vi "GuiUpdate.vi"(7 "GuiRef":T1, 8 "error in":errorcluster, 9 "States":T2=enum."PostUUT") -> (0 "error out":errorcluster, 1 "GuiRefOut":T1, 2 "PASS/FAIL":bool)   [LabVIEW 2013]
uses:
  Ctl/States.ctl
  Ctl/LEDState.ctl
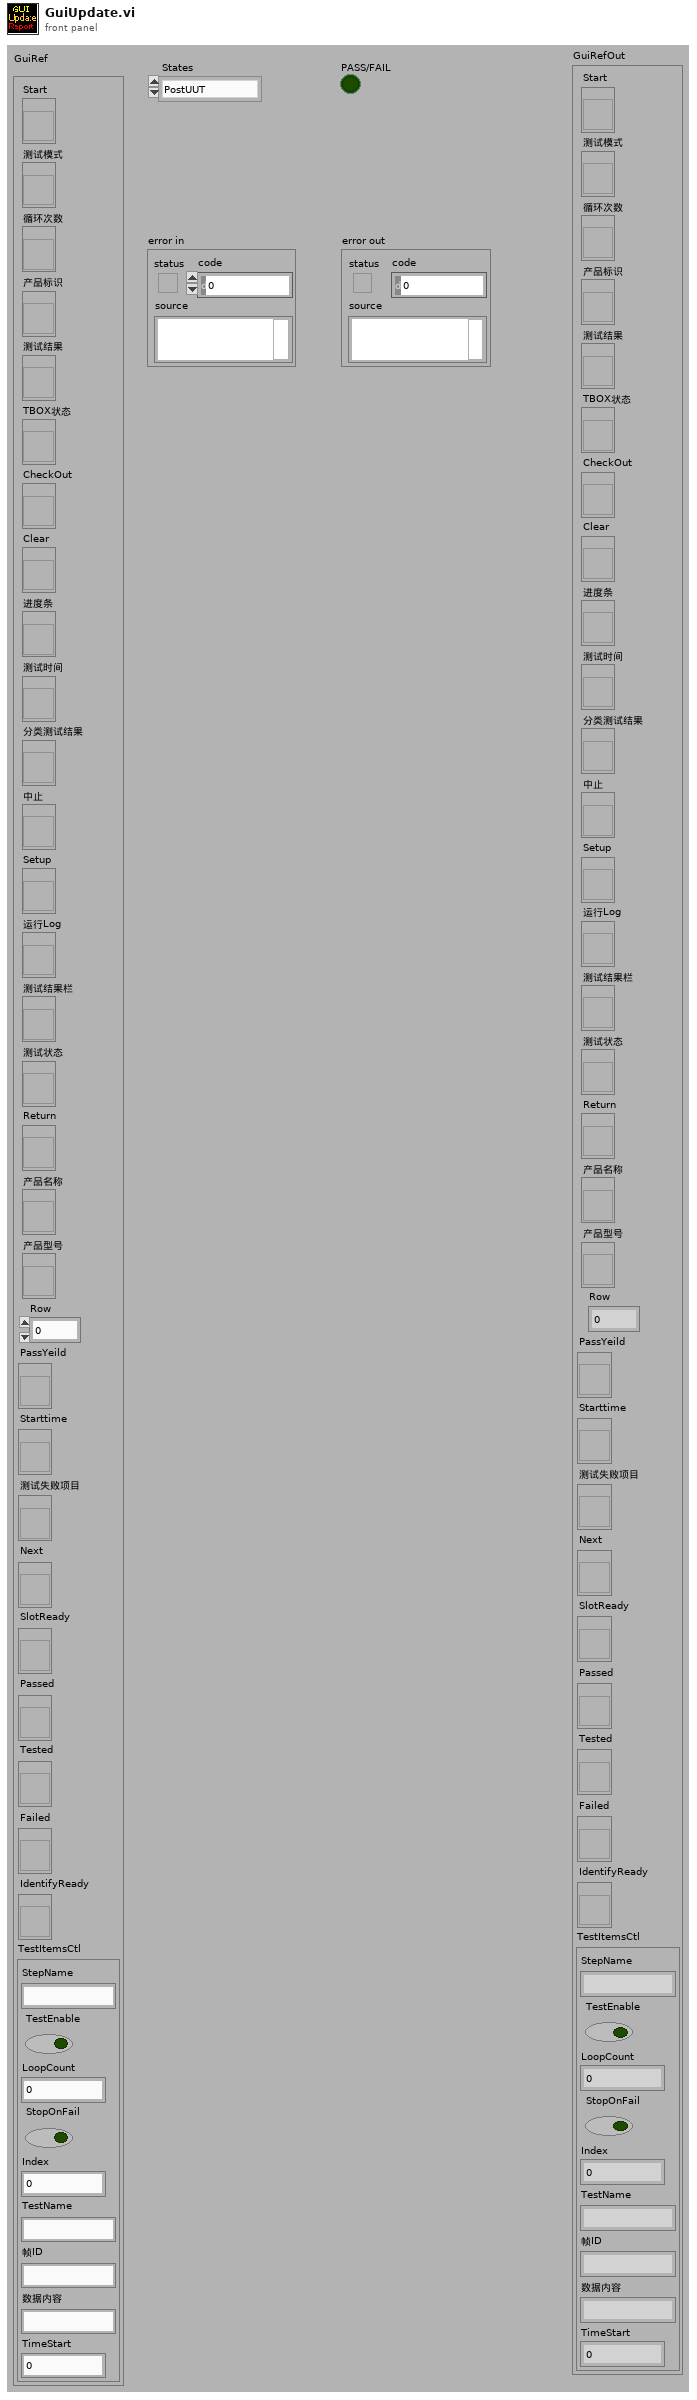
[diagram p1: front panel]
types:
  T1 = typedef "控件.ctl" = cluster{"Start":refnum<vi>, "测试模式":refnum<vi>, "循环次数":refnum<vi>, "产品标识":refnum<vi>, "测试结果":refnum<vi>, "TBOX状态":refnum<vi>, "CheckOut":refnum<vi>, "Clear":refnum<vi>, "进度条":refnum<vi>, "测试时间":refnum<vi>, "分类测试结果":refnum<vi>, "中止":refnum<vi>, "Setup":refnum<vi>, "运行Log":refnum<vi>, "测试结果栏":refnum<vi>, "测试状态":refnum<vi>, "Return":refnum<vi>, "产品名称":refnum<vi>, "产品型号":refnum<vi>, "Row":i32, "PassYeild":refnum<vi>, "Starttime":refnum<vi>, "测试失败项目":refnum<vi>, "Next":refnum<vi>, "SlotReady":refnum<vi>, "Passed":refnum<vi>, "Tested":refnum<vi>, "Failed":refnum<vi>, "IdentifyReady":refnum<vi>, "TestItemsCtl":cluster{"StepName":string, "TestEnable":bool, "LoopCount":u32, "StopOnFail":bool, "Index":u32, "TestName":string, "帧ID":string, "数据内容":string, "TimeStart":u32}}
  T2 = typedef "States.ctl" = enum16{"Init", "PreUUT", "Idle", "SetUp", "TestSequence", "PostUUT", "StopTest", "Debug Mode", "Selection Mode", "Loop Mode", "Error", "Wait"}
  T3 = enum8{"Enabled", "Disabled", "Disabled and Grayed Out"}
  T4 = typedef "LEDState.ctl" = enum16{"默认", "闪烁", "停止闪烁", "真", "假"}
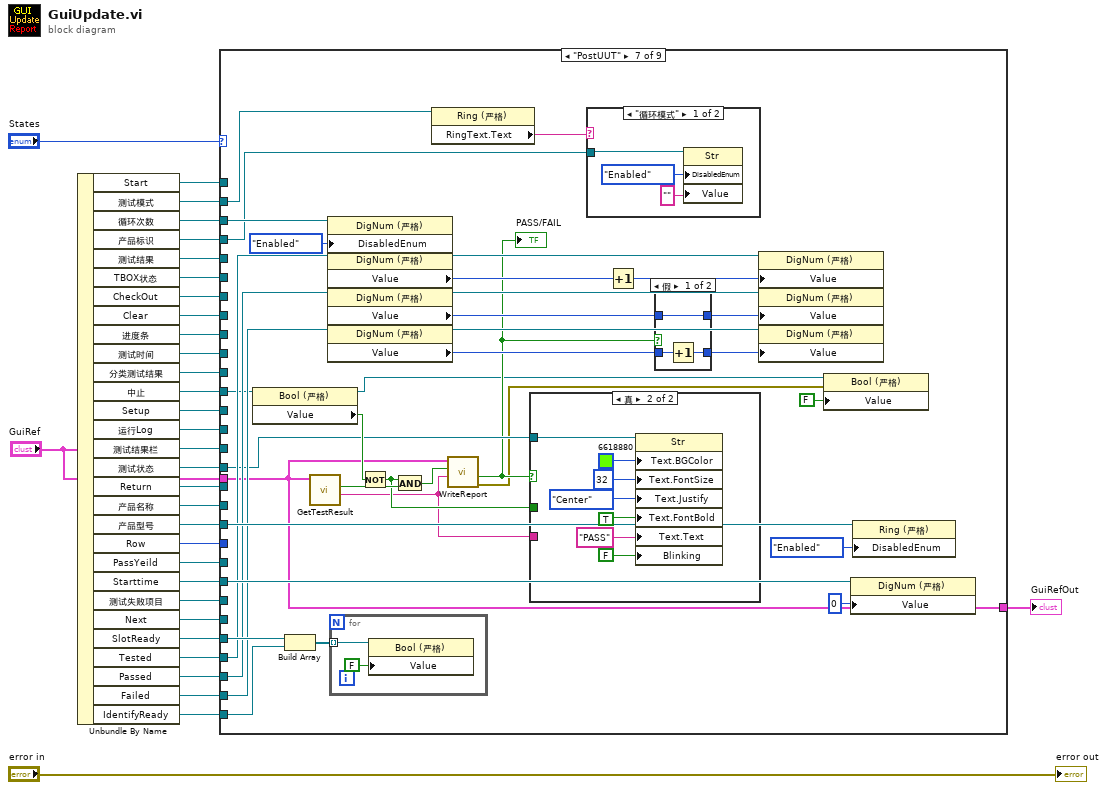
[diagram p0: block diagram]
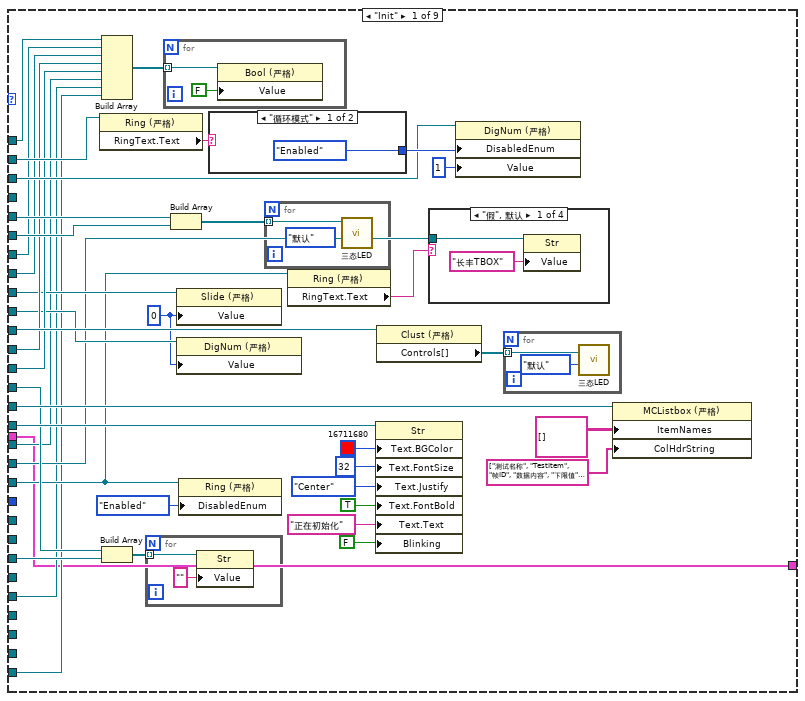
[diagram p2: hidden frame]
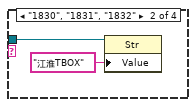
[diagram p3: hidden frame]
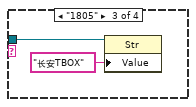
[diagram p4: hidden frame]
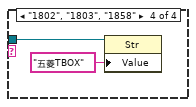
[diagram p5: hidden frame]
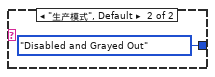
[diagram p6: hidden frame]
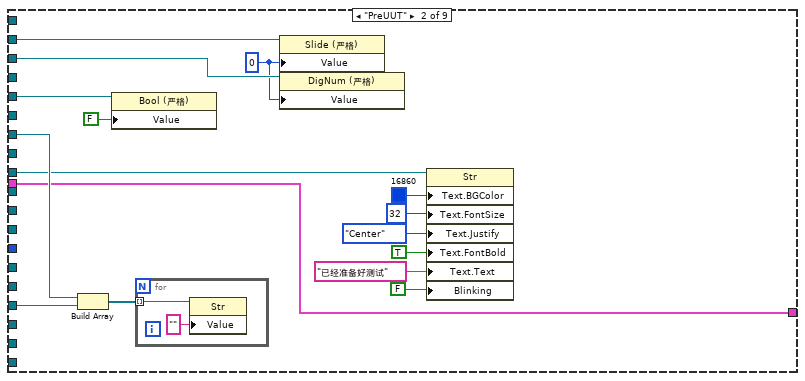
[diagram p7: hidden frame]
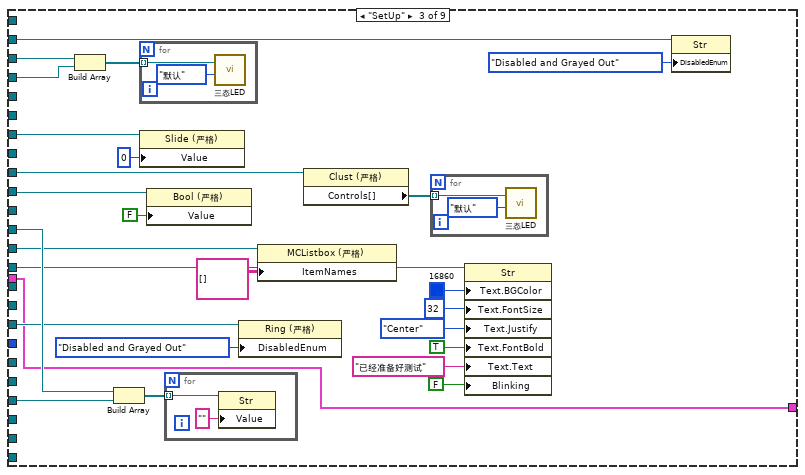
[diagram p8: hidden frame]
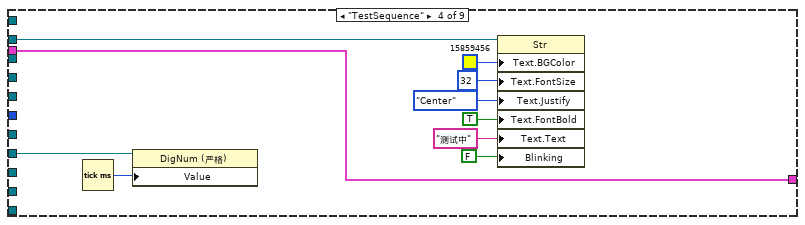
[diagram p9: hidden frame]
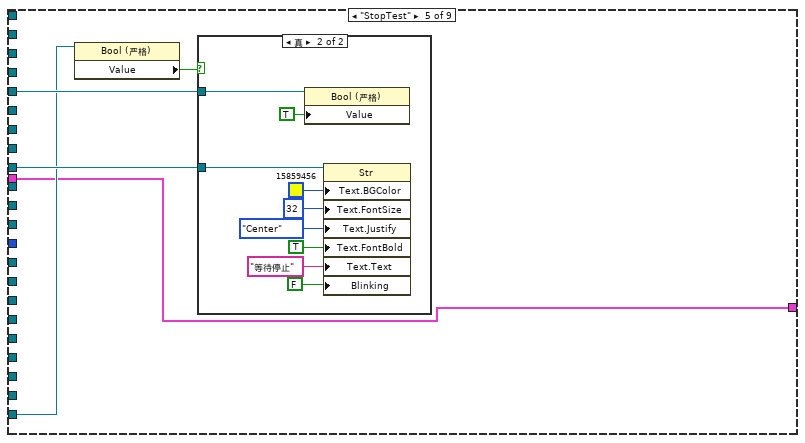
[diagram p10: hidden frame]
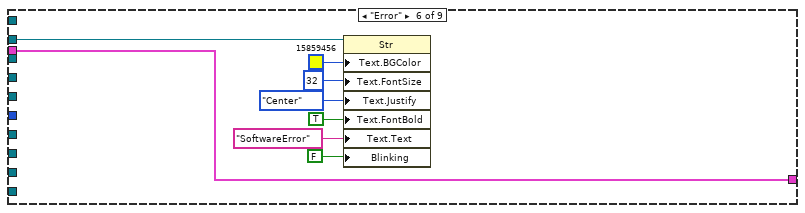
[diagram p12: hidden frame]
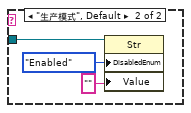
[diagram p13: hidden frame]
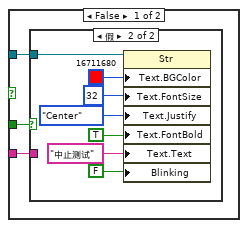
[diagram p14: hidden frame]
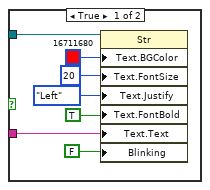
[diagram p15: hidden frame]
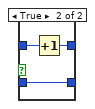
[diagram p16: hidden frame]
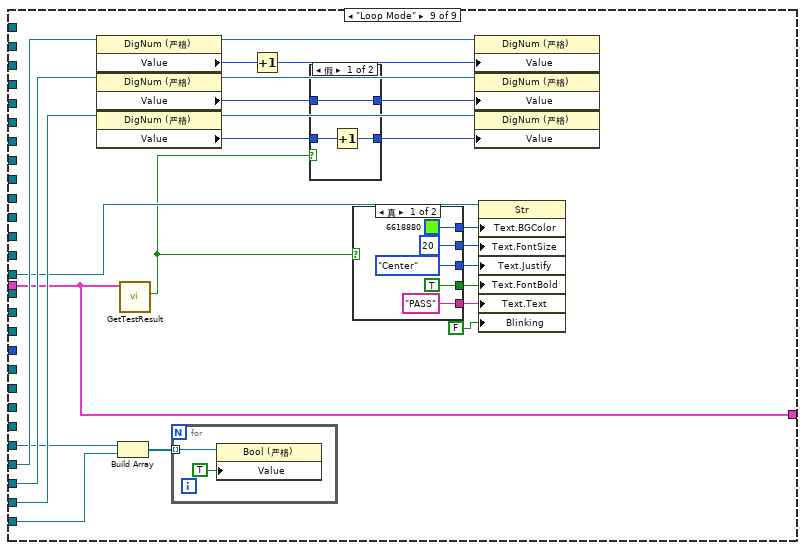
[diagram p18: hidden frame]
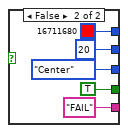
[diagram p19: hidden frame]
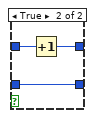
[diagram p20: hidden frame]
diagram:
  n1 = Unbundle By Name("GuiRef") -> ("Start"=w31:refnum<vi>, "测试模式"=w30:refnum<vi>, "循环次数"=w29:refnum<vi>, "产品标识"=w28:refnum<vi>, "测试结果"=w27:refnum<vi>, "TBOX状态"=w26:refnum<vi>, "CheckOut"=w25:refnum<vi>, "Clear"=w24:refnum<vi>, "进度条"=w23:refnum<vi>, "测试时间"=w22:refnum<vi>, "分类测试结果"=w21:refnum<vi>, "中止"=w2:refnum<vi>, "Setup"=w20:refnum<vi>, "运行Log"=w19:refnum<vi>, "测试结果栏"=w18:refnum<vi>, "测试状态"=w17:refnum<vi>, "Return"=w16:refnum<vi>, "产品名称"=w15:refnum<vi>, "产品型号"=w14:refnum<vi>, "Row"=w13:i32, "PassYeild"=w12:refnum<vi>, "Starttime"=w11:refnum<vi>, "测试失败项目"=w10:refnum<vi>, "Next"=w9:refnum<vi>, "SlotReady"=w8:refnum<vi>, "Tested"=w7:refnum<vi>, "Passed"=w6:refnum<vi>, "Failed"=w5:refnum<vi>, "IdentifyReady"=w3:refnum<vi>)
  n2 = case shown="\"PostUUT\"" "States" {
    tunnel: w31 -> [w63 _ _ _ _ _ _ _ _]
    tunnel: w30 -> [w73 _ _ _ _ _ w180 _ _]
    tunnel: w29 -> [w70 _ _ _ _ _ w208 _ _]
    tunnel: w28 -> [_ _ w123 _ _ _ w178 _ _]
    tunnel: w27 -> [w66 _ w115 _ _ _ _ _ _]
    tunnel: w26 -> [w65 _ w114 _ _ _ _ _ _]
    tunnel: w25 -> [w62 _ _ _ _ _ _ _ _]
    tunnel: w24 -> [w61 _ _ _ _ _ _ _ _]
    tunnel: w23 -> [w57 w95 w119 _ _ _ _ _ _]
    tunnel: w22 -> [w56 w94 _ _ _ _ _ _ _]
    tunnel: w21 -> [w68 _ w116 _ _ _ _ _ _]
    tunnel: w20 -> [w59 _ _ _ _ _ _ _ _]
    tunnel: w19 -> [w44 w107 w133 _ _ _ _ _ _]
    tunnel: w18 -> [w54 _ w121 _ _ _ _ _ _]
    tunnel: w17 -> [w51 w98 w126 w145 w155 w167 w187 _ w255]
    tunnel: w16 -> [w35 _ _ _ _ _ _ _ _]
    tunnel: w15 -> [w40 _ _ _ _ _ _ _ _]
    tunnel: w14 -> [w39 _ w124 _ _ _ w204 _ _]
    tunnel: w13 -> [_ _ _ _ _ _ _ _ _]
    tunnel: w12 -> [_ _ _ _ _ _ _ _ _]
    tunnel: w11 -> [_ _ _ w144 _ _ w206 _ _]
    tunnel: w10 -> [w43 w106 w134 _ _ _ _ _ _]
    tunnel: w9 -> [_ _ _ _ _ _ _ _ _]
    tunnel: w8 -> [w37 _ _ _ _ _ w209 _ w252]
    tunnel: w7 -> [_ _ _ _ _ _ w202 _ w272]
    tunnel: w6 -> [_ _ _ _ _ _ w201 _ w259]
    tunnel: w5 -> [_ _ _ _ _ _ w200 _ w258]
    tunnel: "GuiRef" -> [w34 w92 w110 w142 w152 w166 w174 w248 w249]
    tunnel: w3 -> [w36 _ _ _ w153 _ w176 _ w250]
    tunnel: w2 -> [w60 w97 w112 _ w156 _ w175 _ _]
    tunnel: [w34 w92 w110 w142 w152 w166 w174 w248 w249] -> w1
    frame "Init" {
      w55 = 0 ("值")
      n3 = property class="Ring (严格)"(reference=w73) -> ("RingText.Text"=w72:string)  [unwired: 1 in, 2 out]
      n4 = Build Array(w63, w62, w61, w60, w59, w35, w37, w36) -> (w58:refnum<vi>[])
      n5 = Build Array(w44, w43) -> (w42:refnum<vi>[])
      n6 = for {
        tunnel: w42 -> [w83] mode=indexing
        n7 = property class="Str"(reference=w83, "Value"="" ("值")) -> ()  [unwired: 1 in, 2 out]
      }
      n8 = for {
        tunnel: w58 -> [w84] mode=indexing
        n9 = property class="Bool (严格)"(reference=w84, "Value"=FALSE) -> ()  [unwired: 1 in, 2 out]
      }
      n10 = Build Array(w66, w65) -> (w64:refnum<vi>[])
      n11 = property class="Slide (严格)"(reference=w57, "Value"=w55) -> ()  [unwired: 1 in, 2 out]
      n12 = property class="DigNum (严格)"(reference=w56, "Value"=w55) -> ()  [unwired: 1 in, 2 out]
      n13 = property class="Ring (严格)"(reference=w39, "DisabledEnum"=T3."Enabled" ("禁用")) -> ()  [unwired: 1 in, 2 out]
      n14 = case shown="\"循环模式\"" w72 {
        tunnel: [T3."Enabled" ("禁用") T3."Disabled and Grayed Out" ("禁用")] -> w71
        frame "循环模式" {
        }
        frame "生产模式", Default {
        }
      }
      n15 = for {
        tunnel: w64 -> [w86] mode=indexing
        n16 = call "三态LED.vi"("State"=LEDState."默认", "Ctl引用句柄"=w86) -> ()  [unwired: 4 in, 2 out]
      }
      n17 = property class="Ring (严格)"(reference=w39) -> ("RingText.Text"=w38:string)  [unwired: 1 in, 2 out]
      n18 = property class="Str"(reference=w51, "Text.BGColor"=u32 16711680, "Text.FontSize"=32 ("值"), "Text.Justify"=enum16{"Left", "Center", "Right"}."Center" ("文本.调整"), "Text.FontBold"=TRUE ("文本.字体:粗体"), "Text.Text"="正在初始化" ("文本.文本"), "Blinking"=FALSE ("文本.字体:粗体")) -> ()  [unwired: 1 in, 2 out]
      n19 = property class="Clust (严格)"(reference=w68) -> ("Controls[]"=w67:refnum<vi>[])  [unwired: 1 in, 2 out]
      n20 = case shown="\"假\", 默认" w38 {
        tunnel: w40 -> [w74 w77 w79 w81]
        frame "假", Default {
          n21 = property class="Str"(reference=w74, "Value"="长丰TBOX" ("值")) -> ()  [unwired: 1 in, 2 out]
        }
        frame "1830", "1831", "1832" {
          n22 = property class="Str"(reference=w77, "Value"="江淮TBOX" ("值")) -> ()  [unwired: 1 in, 2 out]
        }
        frame "1805" {
          n23 = property class="Str"(reference=w79, "Value"="长安TBOX" ("值")) -> ()  [unwired: 1 in, 2 out]
        }
        frame "1802", "1803", "1858" {
          n24 = property class="Str"(reference=w81, "Value"="五菱TBOX" ("值")) -> ()  [unwired: 1 in, 2 out]
        }
      }
      n25 = property class="DigNum (严格)"(reference=w70, "DisabledEnum"=w71, "Value"=u32 1 ("值")) -> ()  [unwired: 1 in, 2 out]
      n26 = for {
        tunnel: w67 -> [w88] mode=indexing
        n27 = call "三态LED.vi"("State"=LEDState."默认", "Ctl引用句柄"=w88) -> ()  [unwired: 4 in, 2 out]
      }
      n28 = property class="MCListbox (严格)"(reference=w54, "ItemNames"=string[][] [] ("项名"), "ColHdrString"=string[] ["测试名称", "TestItem", "帧ID", "数据内容", "下限值", "上限值", "单位", "间隔时间", "测量值", "结果", "测试时间", "备注", "测试项目"] ("列首字符串[]")) -> ()  [unwired: 1 in, 2 out]
    }
    frame "PreUUT" {
      w93 = 0
      n29 = Build Array(w107, w106) -> (w105:refnum<vi>[])
      n30 = property class="Bool (严格)"(reference=w97, "Value"=FALSE ("值")) -> ()  [unwired: 1 in, 2 out]
      n31 = for {
        tunnel: w105 -> [w109] mode=indexing
        n32 = property class="Str"(reference=w109, "Value"="" ("值")) -> ()  [unwired: 1 in, 2 out]
      }
      n33 = property class="Slide (严格)"(reference=w95, "Value"=w93) -> ()  [unwired: 1 in, 2 out]
      n34 = property class="DigNum (严格)"(reference=w94, "Value"=w93) -> ()  [unwired: 1 in, 2 out]
      n35 = property class="Str"(reference=w98, "Text.BGColor"=u32 16860, "Text.FontSize"=32 ("值"), "Text.Justify"=enum16{"Left", "Center", "Right"}."Center" ("文本.调整"), "Text.FontBold"=TRUE ("文本.字体:粗体"), "Text.Text"="已经准备好测试" ("文本.文本"), "Blinking"=FALSE ("文本.字体:粗体")) -> ()  [unwired: 1 in, 2 out]
    }
    frame "SetUp" {
      n36 = Build Array(w115, w114) -> (w113:refnum<vi>[])
      n37 = Build Array(w133, w134) -> (w135:refnum<vi>[])
      n38 = for {
        tunnel: w113 -> [w136] mode=indexing
        n39 = call "三态LED.vi"("State"=LEDState."默认", "Ctl引用句柄"=w136) -> ()  [unwired: 4 in, 2 out]
      }
      n40 = property class="Slide (严格)"(reference=w119, "Value"=0 ("值")) -> ()  [unwired: 1 in, 2 out]
      n41 = property class="Bool (严格)"(reference=w112, "Value"=FALSE ("值")) -> ()  [unwired: 1 in, 2 out]
      n42 = for {
        tunnel: w135 -> [w141] mode=indexing
        n43 = property class="Str"(reference=w141, "Value"="" ("值")) -> ()  [unwired: 1 in, 2 out]
      }
      n44 = property class="Ring (严格)"(reference=w124, "DisabledEnum"=T3."Disabled and Grayed Out" ("禁用")) -> ()  [unwired: 1 in, 2 out]
      n45 = property class="MCListbox (严格)"(reference=w121, "ItemNames"=string[][] [] ("项名")) -> ()  [unwired: 1 in, 2 out]
      n46 = property class="Clust (严格)"(reference=w116) -> ("Controls[]"=w117:refnum<vi>[])  [unwired: 1 in, 2 out]
      n47 = for {
        tunnel: w117 -> [w138] mode=indexing
        n48 = call "三态LED.vi"("State"=LEDState."默认", "Ctl引用句柄"=w138) -> ()  [unwired: 4 in, 2 out]
      }
      n49 = property class="Str"(reference=w126, "Text.BGColor"=u32 16860, "Text.FontSize"=32 ("值"), "Text.Justify"=enum16{"Left", "Center", "Right"}."Center" ("文本.调整"), "Text.FontBold"=TRUE ("文本.字体:粗体"), "Text.Text"="已经准备好测试" ("文本.文本"), "Blinking"=FALSE ("文本.字体:粗体")) -> ()  [unwired: 1 in, 2 out]
      n50 = property class="Str"(reference=w123, "DisabledEnum"=T3."Disabled and Grayed Out" ("禁用")) -> ()  [unwired: 1 in, 2 out]
    }
    frame "TestSequence" {
      n51 = Tick Count (ms)() -> (millisecond timer value=w143:u32)
      n52 = property class="DigNum (严格)"(reference=w144, "Value"=w143) -> ()  [unwired: 1 in, 2 out]
      n53 = property class="Str"(reference=w145, "Text.BGColor"=u32 15859456, "Text.FontSize"=32 ("值"), "Text.Justify"=enum16{"Left", "Center", "Right"}."Center" ("文本.调整"), "Text.FontBold"=TRUE ("文本.字体:粗体"), "Text.Text"="测试中" ("文本.文本"), "Blinking"=FALSE ("文本.字体:粗体")) -> ()  [unwired: 1 in, 2 out]
    }
    frame "StopTest" {
      n54 = property class="Bool (严格)"(reference=w153) -> ("Value"=w154:bool)  [unwired: 1 in, 2 out]
      n55 = case shown="真" w154 {
        tunnel: w156 -> [_ w165]
        tunnel: w155 -> [_ w157]
        frame False {
        }
        frame True {
          n56 = property class="Bool (严格)"(reference=w165, "Value"=TRUE) -> ()  [unwired: 1 in, 2 out]
          n57 = property class="Str"(reference=w157, "Text.BGColor"=u32 15859456, "Text.FontSize"=32 ("值"), "Text.Justify"=enum16{"Left", "Center", "Right"}."Center" ("文本.调整"), "Text.FontBold"=TRUE ("文本.字体:粗体"), "Text.Text"="等待停止" ("文本.文本"), "Blinking"=FALSE ("文本.字体:粗体")) -> ()  [unwired: 1 in, 2 out]
        }
      }
    }
    frame "Error" {
      n58 = property class="Str"(reference=w167, "Text.BGColor"=u32 15859456, "Text.FontSize"=32 ("值"), "Text.Justify"=enum16{"Left", "Center", "Right"}."Center" ("文本.调整"), "Text.FontBold"=TRUE ("文本.字体:粗体"), "Text.Text"="SoftwareError" ("文本.文本"), "Blinking"=FALSE ("文本.字体:粗体")) -> ()  [unwired: 1 in, 2 out]
    }
    frame "PostUUT" {
      n59 = property class="Bool (严格)"(reference=w175) -> (reference out=w182:refnum<vi>, "Value"=w189:bool)  [unwired: 1 in, 1 out]
      n60 = Build Array(w209, w176) -> (w177:refnum<vi>[])
      n61 = call "GetTestResult.vi"("GuiRef"=w174) -> ("FailStep"=w184:string, "PASS/FAIL"=w190:bool)  [unwired: 9 in]
      n62 = property class="DigNum (严格)"(reference=w208, "DisabledEnum"=T3."Enabled" ("禁用")) -> ()  [unwired: 1 in, 2 out]
      n63 = property class="DigNum (严格)"(reference=w202) -> (reference out=w197:refnum<vi>, "Value"=w199:u32)  [unwired: 1 in, 1 out]
      n64 = property class="DigNum (严格)"(reference=w201) -> (reference out=w191:refnum<vi>, "Value"=w196:u32)  [unwired: 1 in, 1 out]
      n65 = property class="DigNum (严格)"(reference=w200) -> (reference out=w192:refnum<vi>, "Value"=w194:u32)  [unwired: 1 in, 1 out]
      n66 = for {
        tunnel: w177 -> [w211] mode=indexing
        n67 = property class="Bool (严格)"(reference=w211, "Value"=FALSE ("值")) -> ()  [unwired: 1 in, 2 out]
      }
      n68 = Not(x=w189) -> (.not. x?=w185:bool)
      n69 = And(x=w185, y=w190) -> (x .and. y?=w188:bool)
      n70 = property class="Ring (严格)"(reference=w180) -> ("RingText.Text"=w179:string)  [unwired: 1 in, 2 out]
      n71 = call "WriteReport.vi"("StepName"=w184, "Pass/Fail"=w188, "输出簇"=w174) -> ("error out"=w183:errorcluster, "DBresult"=w186:bool)  [unwired: 7 in]
      "PASS/FAIL" <- w186
      n72 = case shown="真" w186 {
        tunnel: w187 -> [w220 w241]
        tunnel: w185 -> [w219 _]
        tunnel: w184 -> [w218 _]
        frame False {
          n73 = case shown="假" w219 {
            tunnel: w220 -> [w222 w229]
            tunnel: w218 -> [w221 _]
            frame True {
              n74 = property class="Str"(reference=w222, "Text.BGColor"=u32 16711680, "Text.FontSize"=20 ("值"), "Text.Justify"=enum16{"Left", "Center", "Right"}."Left" ("文本.调整"), "Text.FontBold"=TRUE ("文本.字体:粗体"), "Text.Text"=w221, "Blinking"=FALSE ("文本.字体:粗体")) -> ()  [unwired: 1 in, 2 out]
            }
            frame False {
              n75 = property class="Str"(reference=w229, "Text.BGColor"=u32 16711680, "Text.FontSize"=32 ("值"), "Text.Justify"=enum16{"Left", "Center", "Right"}."Center" ("文本.调整"), "Text.FontBold"=TRUE ("文本.字体:粗体"), "Text.Text"="中止测试" ("文本.文本"), "Blinking"=FALSE ("文本.字体:粗体")) -> ()  [unwired: 1 in, 2 out]
            }
          }
        }
        frame True {
          n76 = property class="Str"(reference=w241, "Text.BGColor"=u32 6618880, "Text.FontSize"=32 ("值"), "Text.Justify"=enum16{"Left", "Center", "Right"}."Center" ("文本.调整"), "Text.FontBold"=TRUE ("文本.字体:粗体"), "Text.Text"="PASS" ("文本.文本"), "Blinking"=FALSE ("文本.字体:粗体")) -> ()  [unwired: 1 in, 2 out]
        }
      }
      n77 = case shown="\"循环模式\"" w179 {
        tunnel: w178 -> [w212 w217]
        frame "循环模式" {
          n78 = property class="Str"(reference=w212, "DisabledEnum"=T3."Enabled" ("禁用"), "Value"="" ("值")) -> ()  [unwired: 1 in, 2 out]
        }
        frame "生产模式", Default {
          n79 = property class="Str"(reference=w217, "DisabledEnum"=T3."Enabled" ("禁用"), "Value"="" ("值")) -> ()  [unwired: 1 in, 2 out]
        }
      }
      n80 = Increment(x=w199) -> (x+1=w198:u32)
      n81 = case shown="假" w186 {
        tunnel: w196 -> [w244 w247]
        tunnel: [w244 w246] -> w195
        tunnel: w194 -> [w243 w245]
        tunnel: [w242 w245] -> w193
        frame False {
          n82 = Increment(x=w243) -> (x+1=w242:u32)
        }
        frame True {
          n83 = Increment(x=w247) -> (x+1=w246:u32)
        }
      }
      n84 = property class="DigNum (严格)"(reference=w197, "Value"=w198) -> ()  [unwired: 1 in, 2 out]
      n85 = property class="DigNum (严格)"(reference=w191, "Value"=w195) -> ()  [unwired: 1 in, 2 out]
      n86 = property class="DigNum (严格)"(reference=w192, "Value"=w193) -> ()  [unwired: 1 in, 2 out]
      n87 = property class="Bool (严格)"(reference=w182, error in=w183, "Value"=FALSE ("值")) -> ()  [unwired: 2 out]
      n88 = property class="DigNum (严格)"(reference=w206, "Value"=u32 0 ("值")) -> ()  [unwired: 1 in, 2 out]
      n89 = property class="Ring (严格)"(reference=w204, "DisabledEnum"=T3."Enabled" ("禁用")) -> ()  [unwired: 1 in, 2 out]
    }
    frame "Wait", Default {
    }
    frame "Loop Mode" {
      n90 = property class="DigNum (严格)"(reference=w272) -> (reference out=w266:refnum<vi>, "Value"=w263:u32)  [unwired: 1 in, 1 out]
      n91 = property class="DigNum (严格)"(reference=w259) -> (reference out=w265:refnum<vi>, "Value"=w256:u32)  [unwired: 1 in, 1 out]
      n92 = property class="DigNum (严格)"(reference=w258) -> (reference out=w264:refnum<vi>, "Value"=w261:u32)  [unwired: 1 in, 1 out]
      n93 = Build Array(w252, w250) -> (w251:refnum<vi>[])
      n94 = call "GetTestResult.vi"("GuiRef"=w249) -> ("PASS/FAIL"=w254:bool)  [unwired: 9 in, 1 out]
      n95 = for {
        tunnel: w251 -> [w274] mode=indexing
        n96 = property class="Bool (严格)"(reference=w274, "Value"=TRUE ("值")) -> ()  [unwired: 1 in, 2 out]
      }
      n97 = Increment(x=w263) -> (x+1=w262:u32)
      n98 = case shown="假" w254 {
        tunnel: w261 -> [w286 w290]
        tunnel: [w285 w290] -> w260
        tunnel: [w287 w288] -> w257
        tunnel: w256 -> [w287 w289]
        frame False {
          n99 = Increment(x=w286) -> (x+1=w285:u32)
        }
        frame True {
          n100 = Increment(x=w289) -> (x+1=w288:u32)
        }
      }
      n101 = case shown="真" w254 {
        tunnel: [u32 6618880 u32 16711680] -> w271
        tunnel: [20 ("值") 20 ("值")] -> w270
        tunnel: [enum16{"Left", "Center", "Right"}."Center" ("文本.调整") enum16{"Left", "Center", "Right"}."Center" ("文本.调整")] -> w269
        tunnel: [TRUE ("文本.字体:粗体") TRUE ("文本.字体:粗体")] -> w268
        tunnel: ["PASS" ("FailStep") "FAIL" ("FailStep")] -> w253
        frame True {
        }
        frame False {
        }
      }
      n102 = property class="DigNum (严格)"(reference=w266, "Value"=w262) -> ()  [unwired: 1 in, 2 out]
      n103 = property class="DigNum (严格)"(reference=w265, "Value"=w257) -> ()  [unwired: 1 in, 2 out]
      n104 = property class="DigNum (严格)"(reference=w264, "Value"=w260) -> ()  [unwired: 1 in, 2 out]
      n105 = property class="Str"(reference=w255, "Text.BGColor"=w271, "Text.FontSize"=w270, "Text.Justify"=w269, "Text.FontBold"=w268, "Text.Text"=w253, "Blinking"=FALSE ("文本.字体:粗体")) -> ()  [unwired: 1 in, 2 out]
    }
  }
  "GuiRefOut" <- w1
  "error out" <- "error in"
